vi "Optimization Selection.vi"(11 "Master Controller in":refnum<class "EMS User Interface.lvclass">) -> ()   [LabVIEW 2018, in "EMS User Interface Actor.lvlib" / "EMS User Interface.lvclass"]
uses:
  EMS User Interface.lvclass
  C:/Users/Administrator/Desktop/FOR GITHUB UPLOAD/LabVIEW EMS/EMS Generic Actor/EMS Generic/EMS Generic.lvclass
  EMS Generic Actor/EMS Generic/EMS Generic.lvclass/EMS Generic.ctl
  EMS Generic Actor/EMS Generic/Accessors - Global Configuration/Read Global Configuration.vi
  EMS Generic Actor/EMS Generic/Accessors - Global Configuration/Update Global Configuration.vi
  EMS Generic Actor/EMS Generic/EMS Generic.lvclass
panel:
  in  "Opt Relative Path":string="External Code\\Python OnGrid Optimization\\linear_generic.py"
  in  "Optimization Model":enum32{"Price", "PV Smoothing", "Custom"}(radio)
  in  "error in":errorcluster
  in  "Cancel":bool
  in  "OK":bool
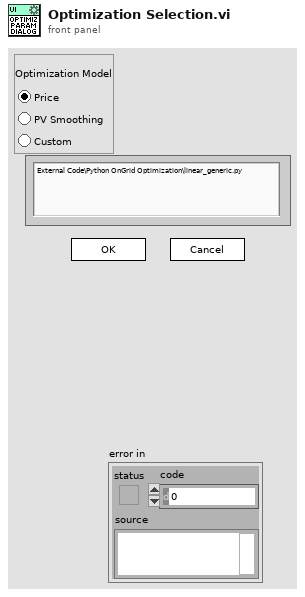
[diagram p1: front panel]
types:
  T1 = enum32{"Invalid", "Standard", "Closed", "Hidden", "Minimized", "Maximized"}
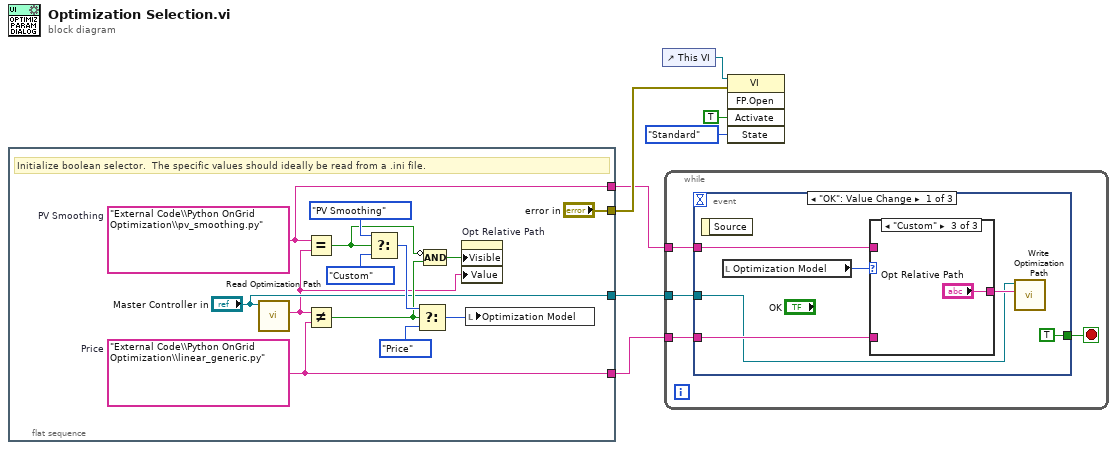
[diagram p0: block diagram]
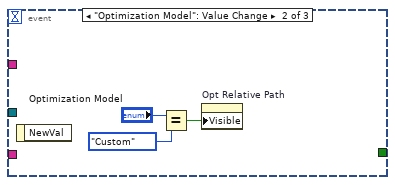
[diagram p4: hidden frame]
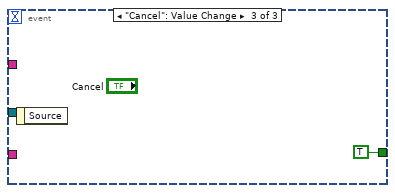
[diagram p5: hidden frame]
diagram:
  n1 = flat-sequence {
    tunnel: ["error in"] -> w4
    tunnel: [w14] -> w2
    tunnel: [w13] -> w3
    tunnel: ["Master Controller in"] -> w1
    frame #0 {
      w14 = "External Code\\Python OnGrid Optimization\\linear_generic.py"  # Price
      w13 = "External Code\\Python OnGrid Optimization\\pv_smoothing.py"  # PV Smoothing
      # "Initialize boolean selector.  The specific values should ideally be read from a .ini file."
      n2 = call "Read Optimization Path.vi"("EMS Generic in"="Master Controller in") -> ("Optimization Relative Path"=w8:string)  [unwired: 8 in, 2 out]
      n3 = Equal?(x=w13, y=w8) -> (x = y?=w12:bool)
      n4 = Not Equal?(x=w8, y=w14) -> (x != y?=w11:bool)
      n5 = Select(t=enum32{"Price", "PV Smoothing", "Custom"}."PV Smoothing" ("Optimization Objective"), s=w12, f=enum32{"Price", "PV Smoothing", "Custom"}."Custom") -> (s? t:f=w19:enum32{"Price", "PV Smoothing", "Custom"})
      n6 = Select(t=w19, s=w11, f=enum32{"Price", "PV Smoothing", "Custom"}."Price") -> (s? t:f=w16:enum32{"Price", "PV Smoothing", "Custom"})
      n7 = Compound Arithmetic op=AND(invert w12, w11) -> (w10:bool)
      n8 = property on="Opt Relative Path" class="Str"("Visible"=w10, "Value"=w8) -> ()  [unwired: 2 in, 2 out]
      n9 = local write "Optimization Model"(w16) -> ()
    }
  }
  n10 = control-ref of="This VI"() -> (w7:refnum<vi>)
  n11 = while {
    tunnel: w3 -> [w23]
    tunnel: w2 -> [w22]
    tunnel: w1 -> [w21]
    stop <- w24 stop-if-true
    n12 = event shown="[0] \"OK\": Value Change" {
      selector: _ -> [_ _ _]
      dyn-events: _ -> [_ _ _]
      timeout: _ -> [_ _ _]
      tunnel: [TRUE ("OK") _ TRUE ("OK")] -> w24
      tunnel: w23 -> [w28 _ _]
      tunnel: w22 -> [w27 _ _]
      tunnel: w21 -> [w25 _ _]
      event "OK": Value Change {
        n13 = event-data() -> ()  [unwired: 1 in, 1 out]
        n14 = local read "Optimization Model"() -> (w29:enum32{"Price", "PV Smoothing", "Custom"})
        n15 = case shown="\"Custom\"" w29 {
          tunnel: [w31 w32 "Opt Relative Path"] -> w26
          tunnel: w28 -> [_ w32 _]
          tunnel: w27 -> [w31 _ _]
          frame "Price", Default {
          }
          frame "PV Smoothing" {
          }
          frame "Custom" {
          }
        }
        n16 = call "Write Optimization Path.vi"("Optimization Path"=w26, "EMS Generic in"=w25) -> ()  [unwired: 8 in, 2 out]
      }
      event "Optimization Model": Value Change {
        n17 = event-data() -> ()  [unwired: 1 in, 1 out]
        n18 = Equal?(x="Optimization Model", y=enum32{"Price", "PV Smoothing", "Custom"}."Custom") -> (x = y?=w35:bool)
        n19 = property on="Opt Relative Path" class="Str"("Visible"=w35) -> ()  [unwired: 2 in, 2 out]
      }
      event "Cancel": Value Change {
        n20 = event-data() -> ()  [unwired: 1 in, 1 out]
      }
    }
  }
  n21 = invoke class="VI" method="FP.Open"(reference=w7, error in=w4, "Activate"=TRUE ("Activate?"), "State"=T1."Standard") -> ()  [unwired: 1 in, 5 out]
